vi "ATF-Log command to DD.vi"(8 "error in (no error)":errorcluster, 11 "Cluster":T1) -> (0 "error out":errorcluster)   [LabVIEW 2022 SP3]
uses:
  Controls/SeCrTs-Notifier ctl.ctl
  Controls/SeCrTs-NS Data type.ctl
  Controls/Commands to Log monitor.ctl
panel:
  in  "Stop 2":bool
  out "value 3":T2
  in  "Server Closed 2":string="The server VI closed the connection."
  out "value 2":T2
  in  "Server Closed":string="The server VI closed the connection."
  in  "Stop":bool
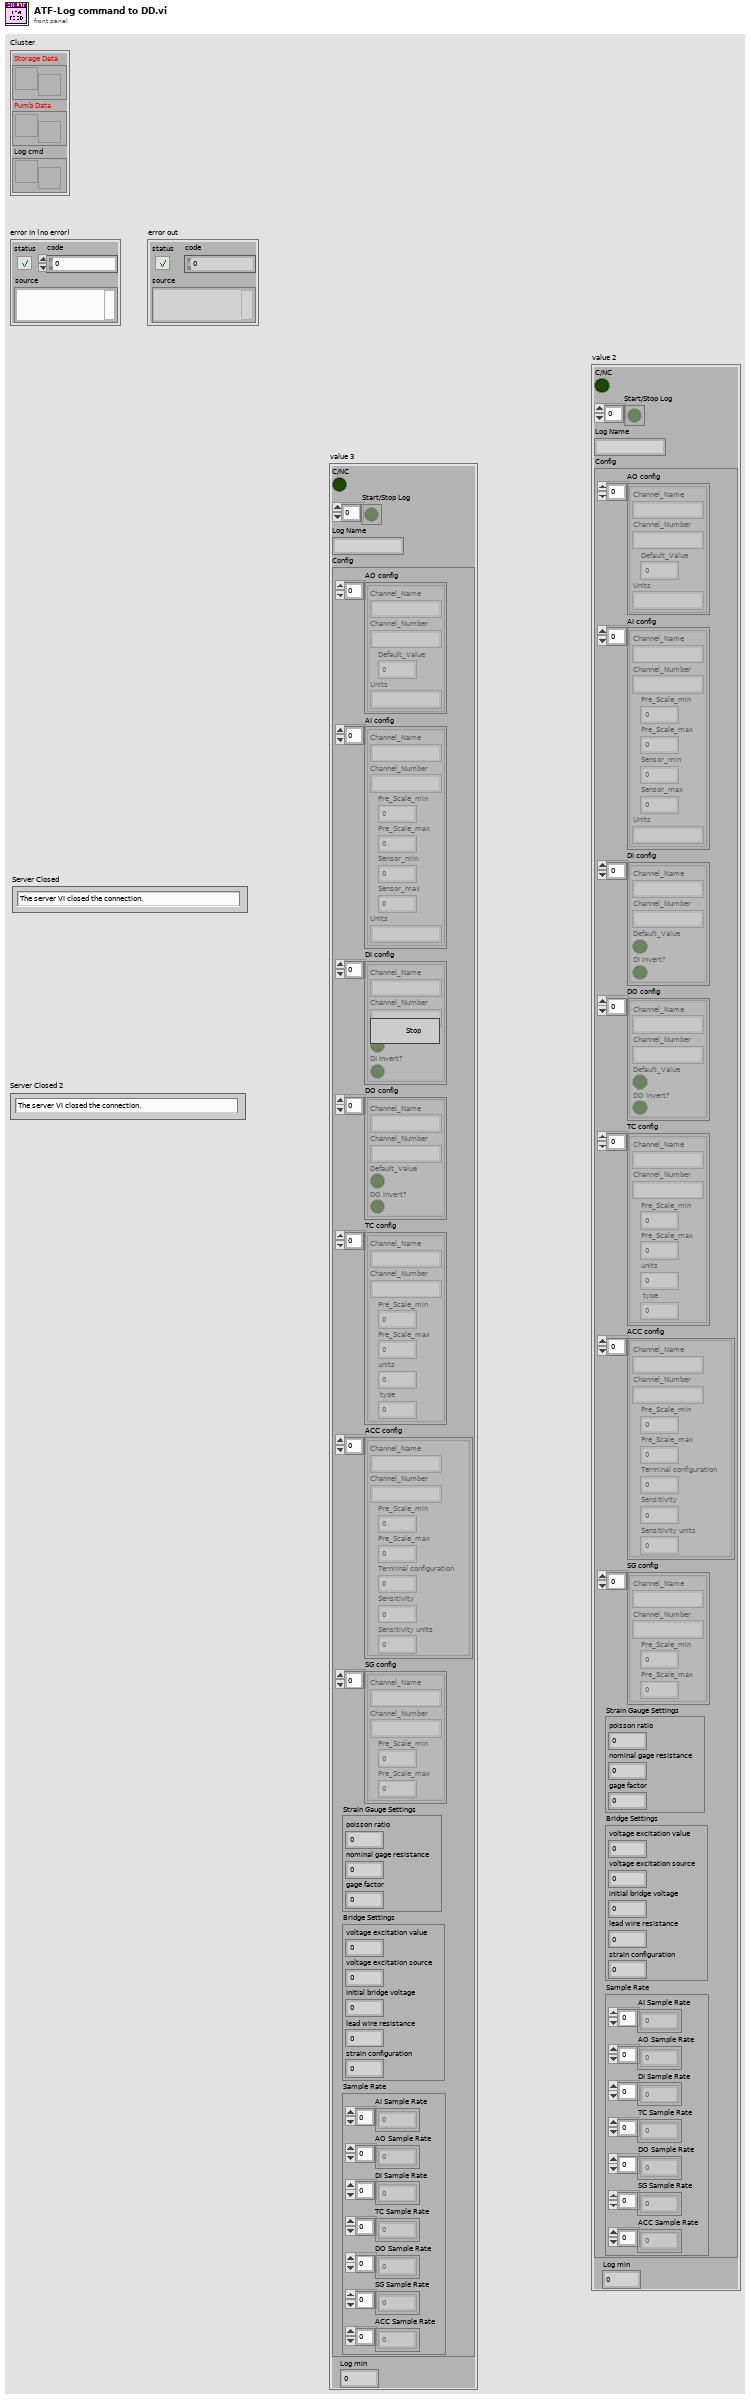
[diagram p1: front panel]
types:
  T1 = typedef "SeCrTs-Notifier ctl.ctl" = cluster{"Storage Data":refnum<notifier>, "Pumb Data":refnum<notifier>, "Log cmd":refnum<notifier>}
  T2 = cluster{"C/NC":bool, "Start/Stop Log":bool[], "Log Name":string, "Config":cluster{"AO config":cluster{"Channel_Name":string, "Channel_Number":string, "Default_Value":dbl, "Units":string}[], "AI config":cluster{"Channel_Name":string, "Channel_Number":string, "Pre_Scale_min":dbl, "Pre_Scale_max":dbl, "Sensor_min":dbl, "Sensor_max":dbl, "Units":string}[], "DI config":cluster{"Channel_Name":string, "Channel_Number":string, "Default_Value":bool, "DI invert?":bool}[], "DO config":cluster{"Channel_Name":string, "Channel_Number":string, "Default_Value":bool, "DO invert?":bool}[], "TC config":cluster{"Channel_Name":string, "Channel_Number":string, "Pre_Scale_min":dbl, "Pre_Scale_max":dbl, "units":i32, " type":i32}[], "ACC config":cluster{"Channel_Name":string, "Channel_Number":string, "Pre_Scale_min":dbl, "Pre_Scale_max":dbl, "Terminal configuration":i32, "Sensitivity":dbl, "Sensitivity units":i32}[], "SG config":cluster{"Channel_Name":string, "Channel_Number":string, "Pre_Scale_min":dbl, "Pre_Scale_max":dbl}[], "Strain Gauge Settings":cluster{"poisson ratio":dbl, "nominal gage resistance":dbl, "gage factor":dbl}, "Bridge Settings":cluster{"voltage excitation value":dbl, "voltage excitation source":i32, "initial bridge voltage":dbl, "lead wire resistance":dbl, "strain configuration":i32}, "Sample Rate":cluster{"AI Sample Rate":dbl[], "AO Sample Rate":dbl[], "DI Sample Rate":dbl[], "TC Sample Rate":dbl[], "DO Sample Rate":dbl[], "SG Sample Rate":dbl[], "ACC Sample Rate":dbl[]}}, "Log min":dbl}
  T3 = cluster{"listener ID":refnum<k5>, "connection ID":refnum<k5>, "Log CMD":refnum<notifier>, "Data":cluster{"C/NC":bool, "Start/Stop Log":bool[], "Log Name":string, "Config":cluster{"AO config":cluster{"Channel_Name":string, "Channel_Number":string, "Default_Value":dbl, "Units":string}[], "AI config":cluster{"Channel_Name":string, "Channel_Number":string, "Pre_Scale_min":dbl, "Pre_Scale_max":dbl, "Sensor_min":dbl, "Sensor_max":dbl, "Units":string}[], "DI config":cluster{"Channel_Name":string, "Channel_Number":string, "Default_Value":bool, "DI invert?":bool}[], "DO config":cluster{"Channel_Name":string, "Channel_Number":string, "Default_Value":bool, "DO invert?":bool}[], "TC config":cluster{"Channel_Name":string, "Channel_Number":string, "Pre_Scale_min":dbl, "Pre_Scale_max":dbl, "units":i32, " type":i32}[], "ACC config":cluster{"Channel_Name":string, "Channel_Number":string, "Pre_Scale_min":dbl, "Pre_Scale_max":dbl, "Terminal configuration":i32, "Sensitivity":dbl, "Sensitivity units":i32}[], "SG config":cluster{"Channel_Name":string, "Channel_Number":string, "Pre_Scale_min":dbl, "Pre_Scale_max":dbl}[], "Strain Gauge Settings":cluster{"poisson ratio":dbl, "nominal gage resistance":dbl, "gage factor":dbl}, "Bridge Settings":cluster{"voltage excitation value":dbl, "voltage excitation source":i32, "initial bridge voltage":dbl, "lead wire resistance":dbl, "strain configuration":i32}, "Sample Rate":cluster{"AI Sample Rate":dbl[], "AO Sample Rate":dbl[], "DI Sample Rate":dbl[], "TC Sample Rate":dbl[], "DO Sample Rate":dbl[], "SG Sample Rate":dbl[], "ACC Sample Rate":dbl[]}}, "Log min":dbl}}
  T4 = typedef "Commands to Log monitor.ctl" = enum16{"initialize", "Close", "Wait on Listener", "Write", "exit"}
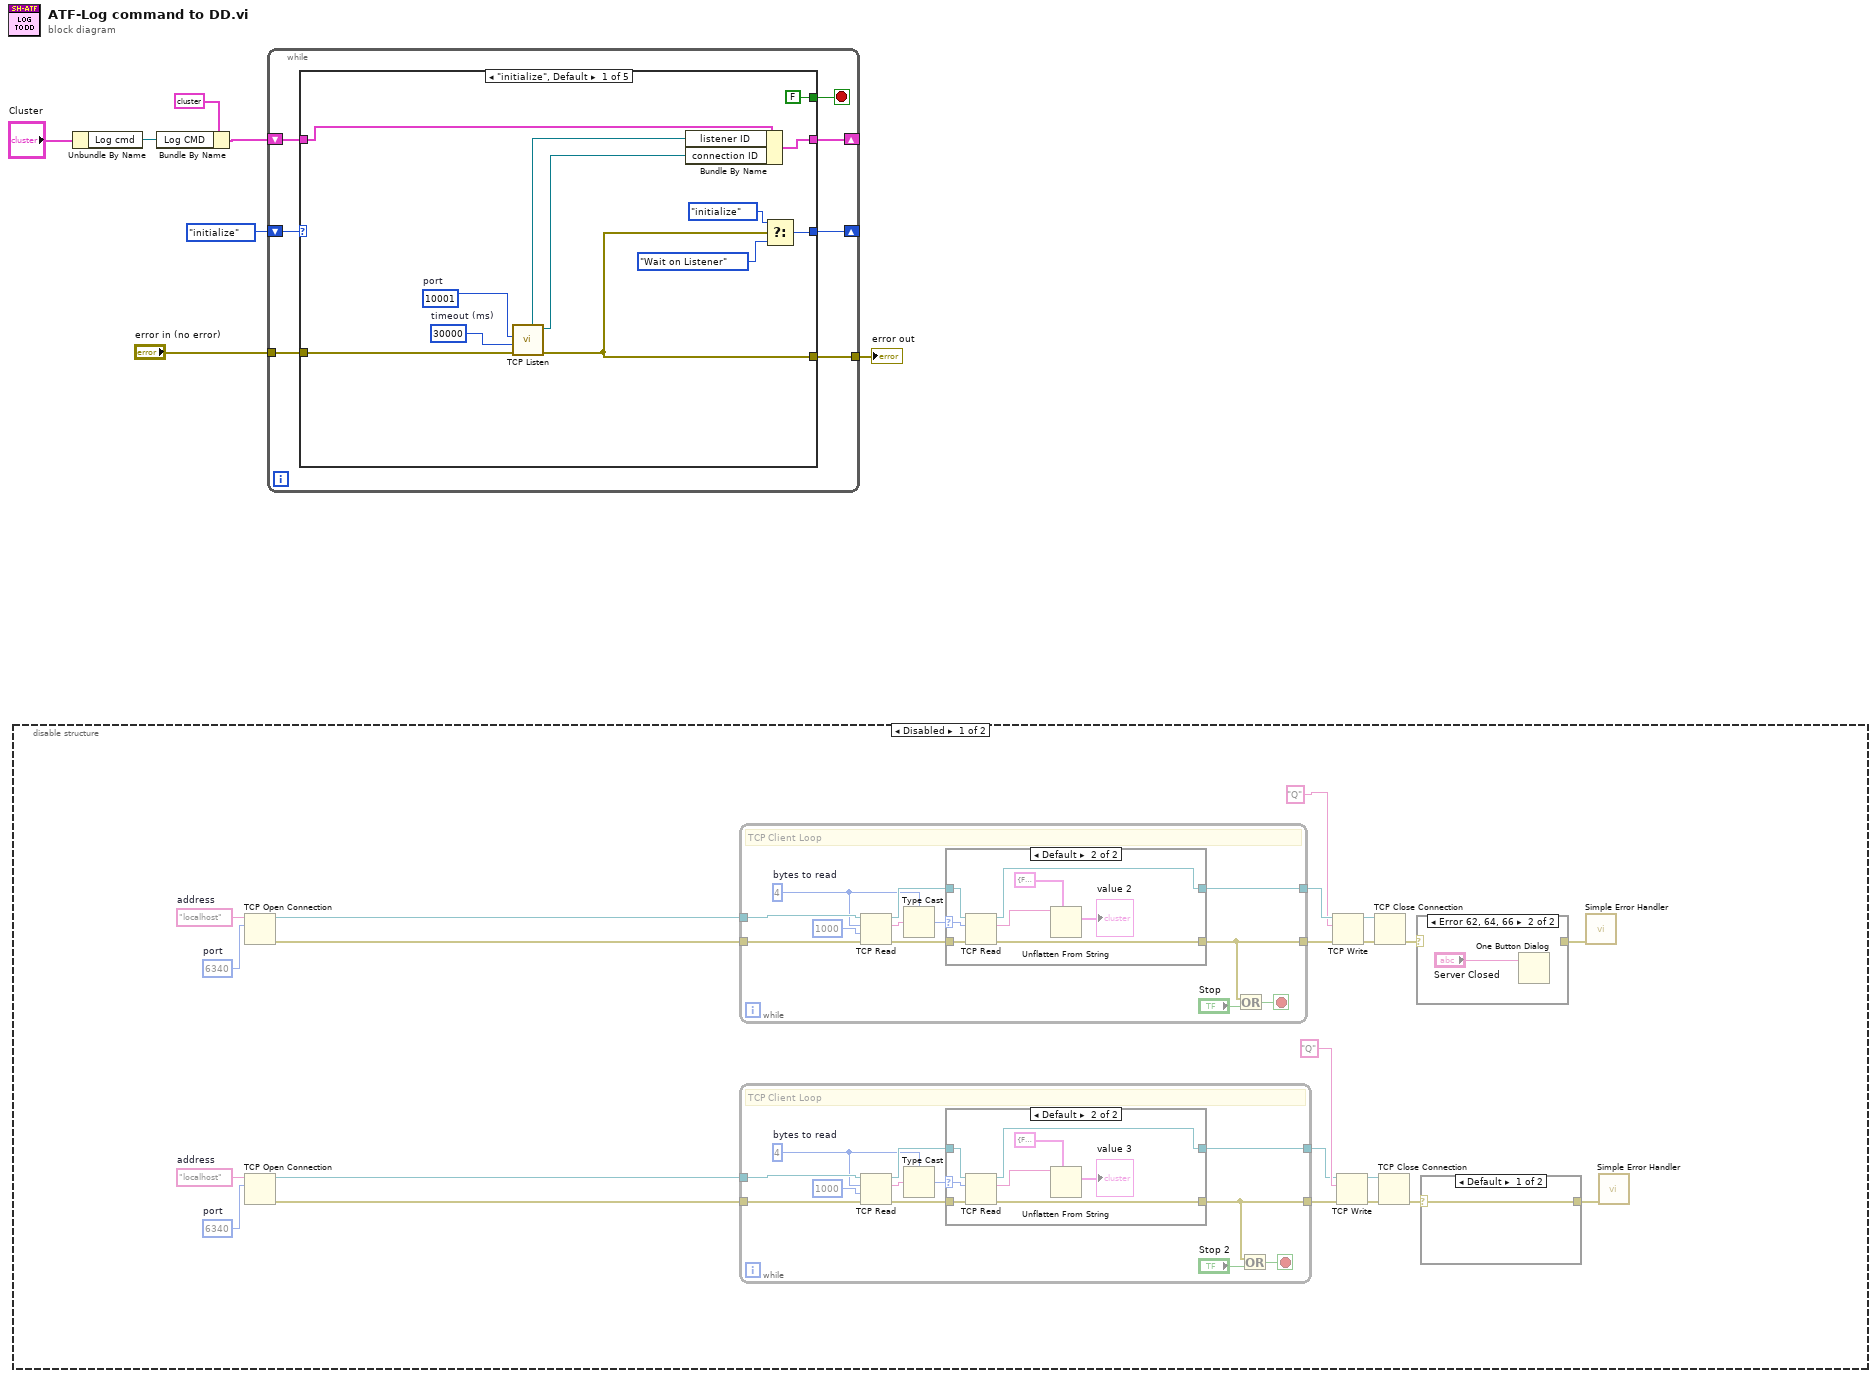
[diagram p0: block diagram]
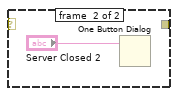
[diagram p2: hidden frame]
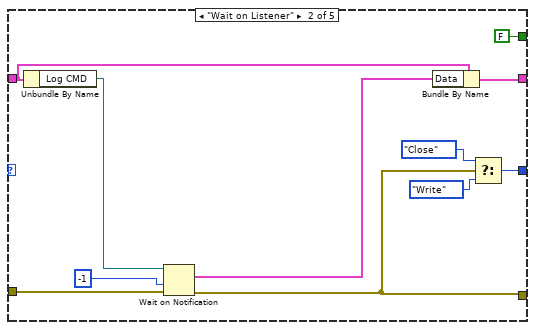
[diagram p7: hidden frame]
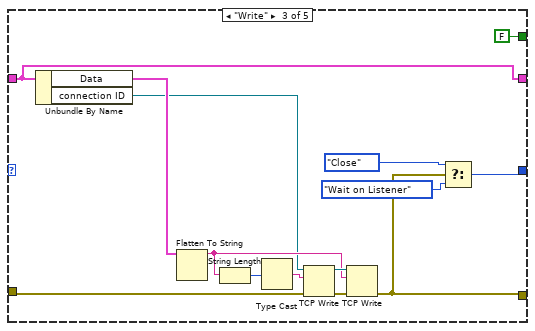
[diagram p8: hidden frame]
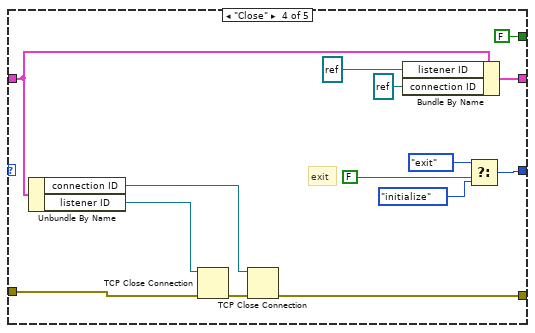
[diagram p9: hidden frame]
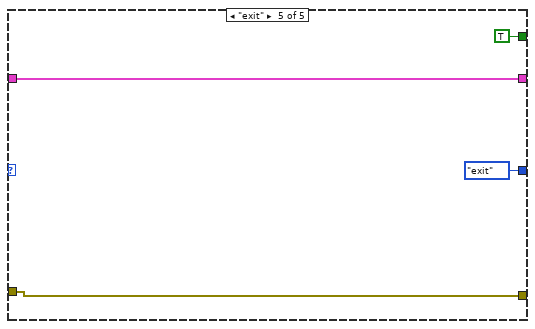
[diagram p10: hidden frame]
diagram:
  n1 = disable-structure shown="Disabled" {
    frame Disabled {
      w20 = u16 6340  # port
      w19 = "localhost"  # address
      w21 = u16 6340  # port
      w22 = "localhost"  # address
      n2 = TCP Open Connection(address=w22, remote port or service name=w21) -> (connection ID=w29:refnum<k5>, error out=w9:errorcluster)  [unwired: 3 in]
      n3 = TCP Open Connection(address=w19, remote port or service name=w20) -> (connection ID=w10:refnum<k5>, error out=w11:errorcluster)  [unwired: 3 in]
      n4 = while {
        tunnel: w9 -> [w63]
        tunnel: w29 -> [w64]
        tunnel: [w59] -> w27
        tunnel: [w58] -> w25
        stop <- w60 stop-if-true
        w62 = 4  # bytes to read
        # "TCP Client Loop"
        n5 = TCP Read(connection ID=w64, bytes to read=w62, error in (no error)=w63, 9:1000 ("timeout ms (25000)")) -> (connection ID out=w66:refnum<k5>, data out=w67:string, error out=w65:errorcluster)  [unwired: 1 in]
        n6 = Type Cast(type=w62, x=w67) -> (*(type *) &x=w57:i32)
        n7 = case shown="Default" w57 {
          selector: w57 -> [_ w73]
          tunnel: w66 -> [w69 w77]
          tunnel: w65 -> [w68 w76]
          tunnel: [w69 w75] -> w59
          tunnel: [w68 w74] -> w58
          frame ..0 {
            # "The server has not written any data"
          }
          frame Default {
            n8 = TCP Read(connection ID=w77, bytes to read=w73, error in (no error)=w76) -> (connection ID out=w75:refnum<k5>, data out=w72:string, error out=w74:errorcluster)  [unwired: 2 in]
            n9 = Unflatten From String(type=T2 {"C/NC"=FALSE, "Start/Stop Log"=[], "Log Name"="", "Config"={"AO config"=[], "AI config"=[], "DI config"=[], "DO config"=[], "TC config"=[], "ACC config"=[], "SG config"=[], "Strain Gauge Settings"={"poisson ratio"=0.0, "nominal gage resistance"=0.0, "gage factor"=0.0}, "Bridge Settings"={"voltage excitation value"=0.0, "voltage excitation source"=0, "initial bridge voltage"=0.0, "lead wire resistance"=0.0, "strain configuration"=0}, "Sample Rate"={"AI Sample Rate"=[], "AO Sample Rate"=[], "DI Sample Rate"=[], "TC Sample Rate"=[], "DO Sample Rate"=[], "SG Sample Rate"=[], "ACC Sample Rate"=[]}}, "Log min"=0.0} ("Cluster"), binary string=w72) -> (value=→"value 2":T2)  [unwired: 3 in, 2 out]
          }
        }
        n10 = Or(x=w58, y="Stop") -> (x .or. y?=w60:bool)
      }
      n11 = while {
        tunnel: w11 -> [w39]
        tunnel: w10 -> [w40]
        tunnel: [w35] -> w13
        tunnel: [w34] -> w15
        stop <- w36 stop-if-true
        w38 = 4  # bytes to read
        # "TCP Client Loop"
        n12 = TCP Read(connection ID=w40, bytes to read=w38, error in (no error)=w39, 9:1000 ("timeout ms (25000)")) -> (connection ID out=w42:refnum<k5>, data out=w43:string, error out=w41:errorcluster)  [unwired: 1 in]
        n13 = Type Cast(type=w38, x=w43) -> (*(type *) &x=w33:i32)
        n14 = case shown="Default" w33 {
          selector: w33 -> [_ w49]
          tunnel: w42 -> [w45 w53]
          tunnel: w41 -> [w44 w52]
          tunnel: [w45 w51] -> w35
          tunnel: [w44 w50] -> w34
          frame ..0 {
            # "The server has not written any data"
          }
          frame Default {
            n15 = TCP Read(connection ID=w53, bytes to read=w49, error in (no error)=w52) -> (connection ID out=w51:refnum<k5>, data out=w48:string, error out=w50:errorcluster)  [unwired: 2 in]
            n16 = Unflatten From String(type=T2 {"C/NC"=FALSE, "Start/Stop Log"=[], "Log Name"="", "Config"={"AO config"=[], "AI config"=[], "DI config"=[], "DO config"=[], "TC config"=[], "ACC config"=[], "SG config"=[], "Strain Gauge Settings"={"poisson ratio"=0.0, "nominal gage resistance"=0.0, "gage factor"=0.0}, "Bridge Settings"={"voltage excitation value"=0.0, "voltage excitation source"=0, "initial bridge voltage"=0.0, "lead wire resistance"=0.0, "strain configuration"=0}, "Sample Rate"={"AI Sample Rate"=[], "AO Sample Rate"=[], "DI Sample Rate"=[], "TC Sample Rate"=[], "DO Sample Rate"=[], "SG Sample Rate"=[], "ACC Sample Rate"=[]}}, "Log min"=0.0} ("Cluster"), binary string=w48) -> (value=→"value 3":T2)  [unwired: 3 in, 2 out]
          }
        }
        n17 = Or(x=w34, y="Stop 2") -> (x .or. y?=w36:bool)
      }
      n18 = TCP Write(connection ID=w27, data in="Q", error in (no error)=w25) -> (connection ID out=w28:refnum<k5>, error out=w26:errorcluster)  [unwired: 2 out]
      n19 = TCP Write(connection ID=w13, data in="Q", error in (no error)=w15) -> (connection ID out=w12:refnum<k5>, error out=w14:errorcluster)  [unwired: 2 out]
      n20 = TCP Close Connection(connection ID=w28, error in (no error)=w26) -> (error out=w24:errorcluster)  [unwired: 1 in, 1 out]
      n21 = TCP Close Connection(connection ID=w12, error in (no error)=w14) -> (error out=w17:errorcluster)  [unwired: 1 in, 1 out]
      n22 = case shown="Error 62, 64, 66" w24 {
        selector: w24 -> [w54 _]
        tunnel: [w54 _] -> w23
        frame #0 {
        }
        frame #1 {
          n23 = One Button Dialog(message="Server Closed") -> ()  [unwired: 1 in, 1 out]
        }
      }
      n24 = case shown="Default" w17 {
        selector: w17 -> [w30 _]
        tunnel: [w30 _] -> w18
        frame #0 {
        }
        frame #1 {
          n25 = One Button Dialog(message="Server Closed 2") -> ()  [unwired: 1 in, 1 out]
        }
      }
      n26 = call <vilib>:"Simple Error Handler.vi"("error in (no error)"=w23) -> ()  [unwired: 4 in, 5 out]
      n27 = call <vilib>:"Simple Error Handler.vi"("error in (no error)"=w18) -> ()  [unwired: 4 in, 5 out]
    }
    frame Enabled {
    }
  }
  n28 = Unbundle By Name("Cluster") -> ("Log cmd"=w1:refnum<notifier>)
  n29 = Bundle By Name(cluster=T3 {"listener ID"=refnum, "connection ID"=refnum, "Log CMD"=refnum, "Data"={"C/NC"=FALSE, "Start/Stop Log"=[], "Log Name"="", "Config"={"AO config"=[], "AI config"=[], "DI config"=[], "DO config"=[], "TC config"=[], "ACC config"=[], "SG config"=[], "Strain Gauge Settings"={"poisson ratio"=0.0, "nominal gage resistance"=0.0, "gage factor"=0.0}, "Bridge Settings"={"voltage excitation value"=0.0, "voltage excitation source"=0, "initial bridge voltage"=0.0, "lead wire resistance"=0.0, "strain configuration"=0}, "Sample Rate"={"AI Sample Rate"=[], "AO Sample Rate"=[], "DI Sample Rate"=[], "TC Sample Rate"=[], "DO Sample Rate"=[], "SG Sample Rate"=[], "ACC Sample Rate"=[]}}, "Log min"=0.0}}, "Log CMD"=w1) -> (w3:T3)
  n30 = while {
    shift-right: [w82] -> _
    shift-left: Commands_to_Log_monitor."initialize" ("Enum") -> [w84]
    tunnel: "error in (no error)" -> [w81]
    tunnel: [w80] -> w5
    shift-right: [w78] -> _
    shift-left: w3 -> [w79]
    stop <- w83 stop-if-true
    n31 = case shown="\"initialize\", Default" w84 {
      tunnel: [FALSE FALSE FALSE FALSE TRUE] -> w83
      tunnel: [w93 w98 w112 w125 Commands_to_Log_monitor."exit" ("f")] -> w82
      tunnel: w81 -> [w90 w107 w116 w132 w139]
      tunnel: [w89 w97 w115 w130 w139] -> w80
      tunnel: w79 -> [w87 w103 w109 w128 w136]
      tunnel: [w88 w104 w109 w129 w136] -> w78
      frame "initialize", Default {
        w96 = u16 10001  # port
        w95 = 30000  # timeout (ms)
        n32 = call <vilib>:"TCP Listen.vi"("error in (no error)"=w90, "timeout ms (wait forever: -1)"=w95, "port"=w96) -> ("error out"=w89:errorcluster, "connection ID"=w86:refnum<k5>, "listener ID"=w85:refnum<k5>)  [unwired: 4 in, 2 out]
        n33 = Bundle By Name(cluster=w87, "listener ID"=w85, "connection ID"=w86) -> (w88:T3)
        n34 = Select(t=Commands_to_Log_monitor."initialize" ("Enum"), s=w89, f=Commands_to_Log_monitor."Wait on Listener") -> (s? t:f=w93:T4)
      }
      frame "Wait on Listener" {
        n35 = Unbundle By Name(w103) -> ("Log CMD"=w106:refnum<notifier>)
        n36 = Wait on Notification(notifier=w106, timeout in ms (-1)=-1, error in (no error)=w107) -> (notification=w102:T2, error out=w97:errorcluster)  [unwired: 1 in, 2 out]
        n37 = Bundle By Name(cluster=w103, "Data"=w102) -> (w104:T3)
        n38 = Select(t=Commands_to_Log_monitor."Close" ("f"), s=w97, f=Commands_to_Log_monitor."Write") -> (s? t:f=w98:T4)
      }
      frame "Write" {
        n39 = Unbundle By Name(w109) -> ("Data"=w113:T2, "connection ID"=w108:refnum<k5>)
        n40 = Flatten To String(anything=w113) -> (data string=w117:string)  [unwired: 3 in, 2 out]
        n41 = String Length(string=w117) -> (length=w119:i32)
        n42 = Type Cast(x=w119) -> (*(type *) &x=w118:string)  [unwired: 1 out]
        n43 = TCP Write(connection ID=w108, data in=w118, error in (no error)=w116) -> (connection ID out=w121:refnum<k5>, error out=w120:errorcluster)  [unwired: 2 out]
        n44 = TCP Write(connection ID=w121, data in=w117, error in (no error)=w120) -> (error out=w115:errorcluster)  [unwired: 3 out]
        n45 = Select(t=Commands_to_Log_monitor."Close" ("f"), s=w115, f=Commands_to_Log_monitor."Wait on Listener") -> (s? t:f=w112:T4)
      }
      frame "Close" {
        # "exit"
        n46 = Unbundle By Name(w128) -> ("connection ID"=w133:refnum<k5>, "listener ID"=w134:refnum<k5>)
        n47 = TCP Close Connection(connection ID=w134, error in (no error)=w132) -> (error out=w131:errorcluster)  [unwired: 1 in, 1 out]
        n48 = TCP Close Connection(connection ID=w133, error in (no error)=w131) -> (error out=w130:errorcluster)  [unwired: 1 in, 1 out]
        n49 = Bundle By Name(cluster=w128, "listener ID"=refnum<k5> refnum, "connection ID"=refnum<k5> refnum) -> (w129:T3)
        n50 = Select(t=Commands_to_Log_monitor."exit", s=FALSE, f=Commands_to_Log_monitor."initialize") -> (s? t:f=w125:T4)
      }
      frame "exit" {
      }
    }
  }
  "error out" <- w5
